vi "(SubVI) Glimpse Information.vi"(6 "Set GB \n(1 GB = 2^30 Bytes)":dbl format="%#_3g", 8 "Height":u32, 9 "Width":u32, 10 "Data type in":enum16{"U8", "I16"}(ring), 11 "Set Record Frame#":u32) -> (0 "max size of a file (kB)":dbl, 1 "Frame# of one .Glimpse":u32, 2 "# of pre-created file":u16, 3 "Data type out":enum16{"U8", "I16"}(ring), 4 "size of one frame (Bytes)":u32, 5 "Pixel depth":i16)   [LabVIEW 2014]
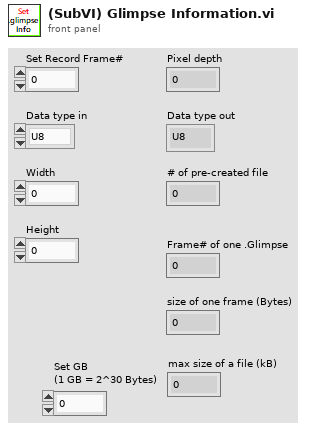
[diagram p1: front panel]
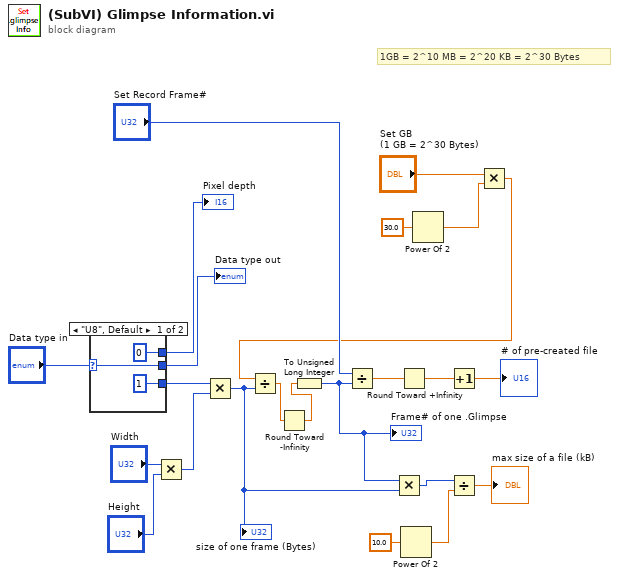
[diagram p0: block diagram]
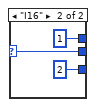
[diagram p2: hidden frame]
diagram:
  # "1GB = 2^10 MB = 2^20 KB = 2^30 Bytes"
  n1 = case shown="\"U8\", Default" "Data type in" {
    selector: "Data type in" -> [w25 w28]
    tunnel: [1 2] -> w16
    tunnel: [w25 w28] -> w18
    tunnel: [i16 0 i16 1] -> w19
    frame "U8", Default {
    }
    frame "I16" {
    }
  }
  "Pixel depth" <- w19
  "Data type out" <- w18
  n2 = Multiply(x="Width", y="Height") -> (x*y=w15:u32)
  n3 = Multiply(x=w16, y=w15) -> (x*y=w5:u32)
  "size of one frame (Bytes)" <- w5
  n4 = Power Of 2(x=10.0) -> (2^x=w2:dbl)
  n5 = Power Of 2(x=30.0) -> (2^x=w10:dbl)
  n6 = Multiply(x="Set GB \n(1 GB = 2^30 Bytes)", y=w10) -> (x*y=w9:dbl)
  n7 = Divide(x=w9, y=w5) -> (x/y=w8:dbl)
  n8 = Round Toward -Infinity(1:w8) -> (0:w7:dbl)
  n9 = To Unsigned Long Integer(number=w7) -> (unsigned 32bit integer=w6:u32)
  "Frame# of one .Glimpse" <- w6
  n10 = Divide(x="Set Record Frame#", y=w6) -> (x/y=w21:dbl)
  n11 = Multiply(x=w6, y=w5) -> (x*y=w4:u32)
  n12 = Round Toward +Infinity(x=w21) -> (ceil(x): smallest int >= x=w22:dbl)
  n13 = Increment(x=w22) -> (x+1=→"# of pre-created file":dbl)
  n14 = Divide(x=w4, y=w2) -> (x/y=→"max size of a file (kB)":dbl)
